vi "SunplusDailyNew.vi"() -> ()   [LabVIEW 2012]
uses:
  <vilib>/addons/database/Auxilliary.llb/DB Tools Cursor Type.ctl
  <vilib>/Utility/NIReport.llb/NI_report.lvclass
  <vilib>/addons/database/Connection.llb/DB Tools Open Connec (Path).vi
  <vilib>/addons/database/Connection.llb/Conn Execute.vi
  <vilib>/addons/database/Recordset.llb/Rec Fetch Recordset Data (R).vi
  <vilib>/addons/database/Recordset.llb/Rec Destroy - Connection.vi
  <vilib>/addons/database/_DB Variant To Data/Database Variant To Data.xnode
  <vilib>/addons/database/NI_Database_API.lvlib
  <vilib>/Utility/NIReport.llb/Excel/NI_Excel.lvclass
  <vilib>/Utility/SMTP/NI_SMTPEmail.lvlib
panel:
  in  "MIME content-type (application/octet-stream)":string="application/octet-stream"
  out "error out 2":errorcluster
  out "error out 4":errorcluster
  in  "?":cluster{"start row":i32, "start column":i32}
  out "error out":errorcluster
  in  "start (0, 0)":cluster{"start row":i32, "start column":i32}
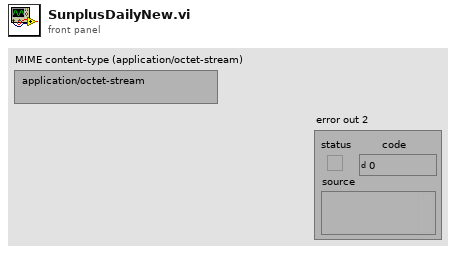
[diagram p1: front panel]
types:
  T1 = typedef "NI_Database_API.lvlib/DB Tools Cursor Type.ctl" = enum16{"forward-only", "keyset", "dynamic", "static"}
  T2 = enum16{"Standard Report", "HTML", "Word", "Excel"}
  T3 = typedef "NI_Database_API.lvlib/Conn ObjectReference.ctl" = refnum<k1>
  T4 = typedef "NI_Database_API.lvlib/Rec ObjectReference.ctl" = refnum<k1>
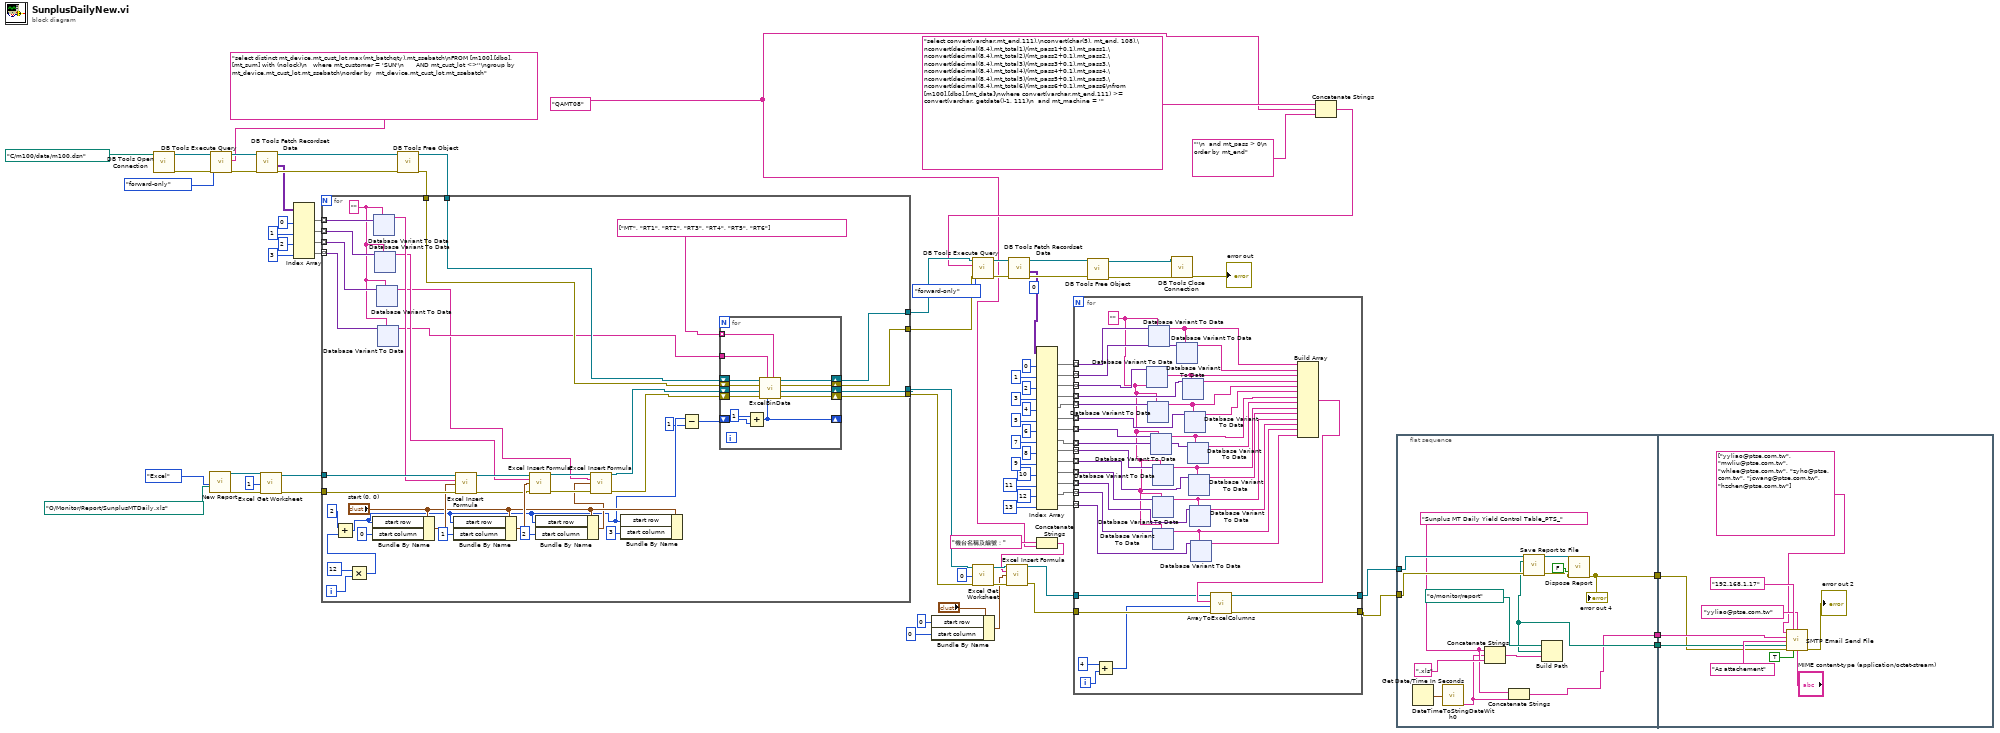
[diagram p0: block diagram]
diagram:
  w7 = "QAMT08" ("Machine")
  (unwired) 0 ("index")
  n1 = call-poly <vilib>:"DB Tools Open Connection.vi"("connection information"=path "C:/m100/data/m100.dsn") -> ("error out"=w83:errorcluster, "connection reference"=w84:T3)  [unwired: 7 in]
  n2 = call <vilib>:"New Report.vi"("report type"=T2."Excel" ("Report Type"), "template (empty)"=path "O:/Monitor/Report/SunplusMTDaily.xls") -> ("report out"=w68:refnum<class "NI_report.lvclass">, "error out"=w67:errorcluster)  [unwired: 12 in]
  n3 = call-poly <vilib>:"DB Tools Execute Query.vi"("error in (no error)"=w83, "cursor type"=DB_Tools_Cursor_Type."forward-only", "SQL query"="select distinct mt_device,mt_cust_lot,max(mt_batchqty),mt_ssebatch\nFROM [m100].[dbo].[mt_sum] with (nolock)\n   where mt_customer = 'SUN'\n      AND mt_cust_lot <>''\ngroup by mt_device,mt_cust_lot,mt_ssebatch\norder by  mt_device,mt_cust_lot,mt_ssebatch", "connection reference"=w84) -> ("error out"=w85:errorcluster, "recordset reference"=w86:T4)  [unwired: 4 in]
  n4 = call-poly <vilib>:"DB Tools Fetch Recordset Data.vi"("error in (no error)"=w85, "recordset reference"=w86) -> ("error out"=w87:errorcluster, "recordset data"=w80:variant[][], "recordset reference out"=w88:T4)  [unwired: 3 in]
  n5 = call <vilib>:"Excel Get Worksheet.vi"("report in"=w68, "worksheet index (0)"=1, "error in (no error)"=w67) -> ("report out"=w64:refnum<class "NI_report.lvclass">, "error out"=w63:errorcluster)  [unwired: 11 in]
  n6 = Index Array(array=w80, index (col) #1=0 ("disabled index (col)"), index (col) #2=1 ("index (col)"), index (col) #3=2 ("index (col)"), index (col) #4=3 ("index (col)")) -> (element #1=w76:variant[], element #2=w75:variant[], element #3=w74:variant[], element #4=w70:variant[])  [unwired: 4 in]
  n7 = call-poly <vilib>:"DB Tools Free Object.vi"("error in (no error)"=w87, "recordset reference"=w88) -> ("error out"=w73:errorcluster, "connection reference"=w72:T3)  [unwired: 8 in]
  n8 = for {
    tunnel: w76 -> [w127] mode=indexing
    tunnel: w75 -> [w126] mode=indexing
    tunnel: w74 -> [w125] mode=indexing
    tunnel: w73 -> [w102]
    tunnel: w72 -> [w103]
    tunnel: w70 -> [w124] mode=indexing
    tunnel: w64 -> [w123]
    tunnel: w63 -> [w122]
    tunnel: [w93] -> w62
    tunnel: [w92] -> w61
    tunnel: [w95] -> w53
    tunnel: [w94] -> w52
    i -> [w106]
    w90 = ""
    n9 = Multiply(x=12, y=w106) -> (x*y=w104:i32)
    n10 = Add(x=2, y=w104) -> (x+y=w99:i32)
    n11 = Bundle By Name(cluster="start (0, 0)", "start row"=w99, "start column"=0) -> (w121:cluster{"start row":i32, "start column":i32})
    n12 = xnode "Database Variant To Data"("database variant"=w127, "type"=w90) -> ("data"=w118:string)  [unwired: 1 in, 1 out]
    n13 = xnode "Database Variant To Data"("database variant"=w126, "type"=w90) -> ("data"=w113:string)  [unwired: 1 in, 1 out]
    n14 = xnode "Database Variant To Data"("database variant"=w125, "type"=w90) -> ("data"=w89:string)  [unwired: 1 in, 1 out]
    n15 = xnode "Database Variant To Data"("database variant"=w124, "type"=w90) -> ("data"=w96:string)  [unwired: 1 in, 1 out]
    n16 = Bundle By Name(cluster="start (0, 0)", "start row"=w99, "start column"=1) -> (w116:cluster{"start row":i32, "start column":i32})
    n17 = call <vilib>:"Excel Insert Formula.vi"("report in"=w123, "formula"=w118, "start (0, 0)"=w121, "error in (no error)"=w122) -> ("report out"=w115:refnum<class "NI_report.lvclass">, "error out"=w114:errorcluster)  [unwired: 10 in]
    n18 = call <vilib>:"Excel Insert Formula.vi"("report in"=w115, "formula"=w113, "start (0, 0)"=w116, "error in (no error)"=w114) -> ("report out"=w111:refnum<class "NI_report.lvclass">, "error out"=w110:errorcluster)  [unwired: 10 in]
    n19 = Bundle By Name(cluster="start (0, 0)", "start row"=w99, "start column"=2) -> (w107:cluster{"start row":i32, "start column":i32})
    n20 = call <vilib>:"Excel Insert Formula.vi"("report in"=w111, "formula"=w89, "start (0, 0)"=w107, "error in (no error)"=w110) -> ("report out"=w101:refnum<class "NI_report.lvclass">, "error out"=w100:errorcluster)  [unwired: 10 in]
    n21 = Bundle By Name(cluster="start (0, 0)", "start row"=w99, "start column"=3) -> ()  [unwired: 1 out]
    n22 = Subtract(x=w99, y=1) -> (x-y=w97:i32)
    n23 = for {
      shift-right: [w139] -> w95
      shift-left: w103 -> [w132]
      shift-right: [w138] -> w94
      shift-left: w102 -> [w131]
      shift-right: [w137] -> w93
      shift-left: w101 -> [w130]
      shift-right: [w136] -> w92
      shift-left: w100 -> [w129]
      shift-right: [w135] -> _
      shift-left: w97 -> [w134]
      tunnel: w96 -> [w133]
      tunnel: string[] ["MT", "RT1", "RT2", "RT3", "RT4", "RT5", "RT6"] ("Array") -> [w128] mode=indexing
      n24 = Add(x=1, y=w134) -> (x+y=w135:i32)
      n25 = call "ExcelBinData.vi"("step"=w128, "start row"=w135, "jobno"=w133, "error in (no error) 2"=w129, "report in"=w130, "error in (no error)"=w131, "connection reference 2"=w132) -> ("error out 2"=w136:errorcluster, "report out"=w137:refnum<class "NI_report.lvclass">, "error out"=w138:errorcluster, "connection reference"=w139:T3)  [unwired: 1 in]
    }
  }
  n26 = Bundle By Name(cluster="?", "start row"=0, "start column"=0) -> (w12:cluster{"start row":i32, "start column":i32})
  n27 = call <vilib>:"Excel Get Worksheet.vi"("report in"=w62, "worksheet index (0)"=0, "error in (no error)"=w61) -> ("report out"=w17:refnum<class "NI_report.lvclass">, "error out"=w16:errorcluster)  [unwired: 11 in]
  n28 = Concatenate Strings("機台名稱及編號：" ("formula"), w7) -> (w9:string)
  n29 = call <vilib>:"Excel Insert Formula.vi"("report in"=w17, "formula"=w9, "start (0, 0)"=w12, "error in (no error)"=w16) -> ("report out"=w11:refnum<class "NI_report.lvclass">, "error out"=w10:errorcluster)  [unwired: 10 in]
  n30 = Concatenate Strings("select convert(varchar,mt_end,111),\nconvert(char(5), mt_end, 108),\nconvert(decimal(8,4),mt_total1)/(mt_pass1+0.1),mt_pass1,\nconvert(decimal(8,4),mt_total2)/(mt_pass2+0.1),mt_pass2,\nconvert(decimal(8,4),mt_total3)/(mt_pass3+0.1),mt_pass3,\nconvert(decimal(8,4),mt_total4)/(mt_pass4+0.1),mt_pass4,\nconvert(decimal(8,4),mt_total5)/(mt_pass5+0.1),mt_pass5,\nconvert(decimal(8,4),mt_total6)/(mt_pass6+0.1),mt_pass6\nfrom [m100].[dbo].[mt_data]\nwhere convert(varchar,mt_end,111) >= convert(varchar, getdate()-1, 111)\n  and mt_machine = '" ("SQL query"), w7, "'\n  and mt_pass > 0\n  order by mt_end" ("SQL query")) -> (w18:string)
  n31 = call-poly <vilib>:"DB Tools Execute Query.vi"("error in (no error)"=w52, "cursor type"=DB_Tools_Cursor_Type."forward-only", "SQL query"=w18, "connection reference"=w53) -> ("error out"=w59:errorcluster, "recordset reference"=w58:T4)  [unwired: 4 in]
  n32 = call-poly <vilib>:"DB Tools Fetch Recordset Data.vi"("error in (no error)"=w59, "recordset reference"=w58) -> ("error out"=w56:errorcluster, "recordset data"=w49:variant[][], "recordset reference out"=w57:T4)  [unwired: 3 in]
  n33 = Index Array(array=w49, index (col) #1=0 ("disabled index (col)"), index (col) #2=1 ("index (col)"), index (col) #3=2 ("index (col)"), index (col) #4=3 ("index (col)"), index (col) #5=4 ("index (col)"), index (col) #6=5 ("index (col)"), index (col) #7=6 ("index (col)"), index (col) #8=7 ("index (col)"), index (col) #9=8 ("index (col)"), index (col) #10=9 ("index (col)"), index (col) #11=10 ("index (col)"), index (col) #12=11 ("index (col)"), index (col) #13=12 ("index (col)"), index (col) #14=13 ("index (col)")) -> (element #1=w46:variant[], element #2=w45:variant[], element #3=w44:variant[], element #4=w33:variant[], element #5=w32:variant[], element #6=w31:variant[], element #7=w30:variant[], element #8=w29:variant[], element #9=w28:variant[], element #10=w27:variant[], element #11=w26:variant[], element #12=w25:variant[], element #13=w22:variant[], element #14=w21:variant[])  [unwired: 14 in]
  n34 = for {
    tunnel: w46 -> [w305] mode=indexing
    tunnel: w45 -> [w304] mode=indexing
    tunnel: w44 -> [w303] mode=indexing
    tunnel: w33 -> [w301] mode=indexing
    tunnel: w32 -> [w297] mode=indexing
    tunnel: w31 -> [w295] mode=indexing
    tunnel: w30 -> [w293] mode=indexing
    tunnel: w29 -> [w290] mode=indexing
    tunnel: w28 -> [w289] mode=indexing
    tunnel: w27 -> [w288] mode=indexing
    tunnel: w26 -> [w285] mode=indexing
    tunnel: w25 -> [w284] mode=indexing
    tunnel: w22 -> [w281] mode=indexing
    tunnel: w21 -> [w280] mode=indexing
    tunnel: w11 -> [w275]
    tunnel: w10 -> [w274]
    tunnel: [w270] -> w6
    tunnel: [w269] -> w5
    i -> [w273]
    w277 = ""
    n35 = Add(x=4, y=w273) -> (x+y=w271:i32)
    n36 = xnode "Database Variant To Data"("database variant"=w303, "type"=w277) -> ("data"=w299:string)  [unwired: 1 in, 1 out]
    n37 = xnode "Database Variant To Data"("database variant"=w297, "type"=w277) -> ("data"=w296:string)  [unwired: 1 in, 1 out]
    n38 = xnode "Database Variant To Data"("database variant"=w305, "type"=w277) -> ("data"=w300:string)  [unwired: 1 in, 1 out]
    n39 = xnode "Database Variant To Data"("database variant"=w293, "type"=w277) -> ("data"=w292:string)  [unwired: 1 in, 1 out]
    n40 = xnode "Database Variant To Data"("database variant"=w289, "type"=w277) -> ("data"=w287:string)  [unwired: 1 in, 1 out]
    n41 = xnode "Database Variant To Data"("database variant"=w285, "type"=w277) -> ("data"=w283:string)  [unwired: 1 in, 1 out]
    n42 = xnode "Database Variant To Data"("database variant"=w281, "type"=w277) -> ("data"=w279:string)  [unwired: 1 in, 1 out]
    n43 = xnode "Database Variant To Data"("database variant"=w304, "type"=w300) -> ("data"=w302:string)  [unwired: 1 in, 1 out]
    n44 = xnode "Database Variant To Data"("database variant"=w301, "type"=w299) -> ("data"=w298:string)  [unwired: 1 in, 1 out]
    n45 = xnode "Database Variant To Data"("database variant"=w295, "type"=w296) -> ("data"=w294:string)  [unwired: 1 in, 1 out]
    n46 = xnode "Database Variant To Data"("database variant"=w290, "type"=w292) -> ("data"=w291:string)  [unwired: 1 in, 1 out]
    n47 = xnode "Database Variant To Data"("database variant"=w288, "type"=w287) -> ("data"=w286:string)  [unwired: 1 in, 1 out]
    n48 = xnode "Database Variant To Data"("database variant"=w284, "type"=w283) -> ("data"=w282:string)  [unwired: 1 in, 1 out]
    n49 = xnode "Database Variant To Data"("database variant"=w280, "type"=w279) -> ("data"=w278:string)  [unwired: 1 in, 1 out]
    n50 = Build Array(w300, w302, w299, w298, w296, w294, w292, w291, w287, w286, w283, w282, w279, w278) -> (w276:string[])
    n51 = call "ArrayToExcelColumns.vi"("error in (no error)"=w274, "start row"=w271, "ArrayData"=w276, "report in"=w275) -> ("error in (no error) 2"=w269:errorcluster, "report in 2"=w270:refnum<class "NI_report.lvclass">)  [unwired: 6 in]
  }
  n52 = call-poly <vilib>:"DB Tools Free Object.vi"("error in (no error)"=w56, "recordset reference"=w57) -> ("error out"=w54:errorcluster, "connection reference"=w55:T3)  [unwired: 8 in]
  n53 = call <vilib>:"DB Tools Close Connection.vi"("error in (no error)"=w54, "connection reference"=w55) -> ("error out"=→"error out":errorcluster)  [unwired: 5 in]
  n54 = flat-sequence {
    tunnel: w6 -> [w763]
    tunnel: w5 -> [w762]
    tunnel: [w754] -> w3
    tunnel: [w758] -> w2
    tunnel: [w757] -> w1
    tunnel: w3 -> [w771]
    tunnel: w2 -> [w770]
    tunnel: w1 -> [w769]
    frame #0 {
      w756 = "Sunplus MT Daily Yield Control Table_PTS_" ("string")
      n55 = Get Date/Time In Seconds() -> (seconds since 1Jan1904=w760:timestamp)
      n56 = call "DateTimeToStringDateWith0.vi"("time stamp"=w760) -> ("Dateyyyymmdd"=w755:string)  [unwired: 9 in, 1 out]
      n57 = Concatenate Strings(w756, w755, ".xls" ("string")) -> (w759:string)
      n58 = Concatenate Strings(w756, w755) -> (w754:string)
      n59 = Build Path(base path=path "o:/monitor/report", name or relative path=w759) -> (appended path=w758:path)
      n60 = call-dynamic "Save Report to File.vi"("report in"=w763, "report file path"=w758, "error in (no error)"=w762) -> ("report out"=w765:refnum<class "NI_report.lvclass">, "error out"=w764:errorcluster)  [unwired: 11 in]
      n61 = call-dynamic "Dispose Report.vi"("report in"=w765, "save changes? (F)"=FALSE, "error in (no error)"=w764) -> ("error out"=w757:errorcluster)  [unwired: 12 in]
      "error out 4" <- w757
    }
    frame #1 {
      n62 = call <vilib>:"SMTP Email Send File.vi"("recipients"=string[] ["yyliao@ptse.com.tw", "mwliu@ptse.com.tw", "whlee@ptse.com.tw", "zyho@ptse.com.tw", "jcwang@ptse.com.tw", "hzchen@ptse.com.tw"], "mail server"="192.168.1.17", "return address"="yyliao@ptse.com.tw", "subject ([No Subject])"=w771, "message"="As attachement", "file path"=w770, "error in (no error)"=w769, "binary? (F)"=TRUE, "MIME content-type (application/octet-stream)"="MIME content-type (application/octet-stream)") -> ("error out"=→"error out 2":errorcluster)  [unwired: 5 in, 1 out]
    }
  }
